vi "GEA_Brute_Force_SM0.vi"() -> ()   [LabVIEW 2009]
uses:
  <vilib>/Instr/_visa.llb/VISA Configure Serial Port (Instr).vi
panel:
  out "ACK":bool
  out "DataReturned":u8[](array[numeric]) format="%.0x"
  out "element":u8
  out "CRCRead":u8[](array[numeric]) format="%.0x"
  out "CRCArray":u8[](array[numeric]) format="%.0x"
  out "CRC Match":bool
  out "States Out":string
  out "error out":errorcluster
  in  "Source Address":u8=128 format="%.0x"
  in  "Command Data":u8[](array[numeric]) format="%02x"
  in  "Destination Address":u8=96 format="%.0x"
  in  "Command":u8(ring)=15 items=["CMD_WRITE_SETPOINTS", "RQST_NON_CRIT_VERSION", "RQST_CRIT_VERSION", "RQST_EEPROM_VERSION", "RQST_T2_RESISTANCE", "RQST_T3A_RESISTANCE", "RQST_T3B_RESISTANCE", "RQST_T4_RESISTANCE", "RQST_T5_RESISTANCE", "RQST_IDLB_RESISTANCE", "RQST_MODE_SELECT_RESISTANCE", "RQST_STATUS INFO", "RQST_SS_FAULT_COUNTS", "RQST_OTHER_FAULT_COUNTS", "CMD_CLEAR_FAULT_COUNTS", "RQST_HYPERTERM_OUTPUT_DATA", "RQST_READ_PERSONALITY", "RQST_DSM_OVERRIDE_STATUS", "RQST_STATUS_QUERY", "RQST_HEM_KWH_DATA", "RQST_SERVICE_ERROR_CODES", "RQST_OVERRIDE_STATUS", "CMD_CLEAR_OVERRIDE_STATUS", "CMD_CLEAR_ENERGY_USAGE_CTRS", "CMD_COMP_OFF", "CMD_UE_2_SECONDS", "CMD_LE_2_SECONDS", "CMD_COMP_ON", "CMD_HP_RUN_6MIN", "RQST_TEMP_RANGE", "RQST_VACATION_RANGE", "RQST_STD_ELEC_RANGE", "RQST_WATER_CAPACITY", "CMD_CANCEL_EEV_POSITION", "RQST_SUPPORTED_MODES", "CMD_CONTROL_FAN1", "CMD_EEV_POSITION", "CMD_SET_EEV_START_POSITION", "CMD_SET_EEV_STOP_POSITION", "CMD_UPDATE_DSM_LEVEL", "CMD_SET_PID_I_DENOMINATOR", "CMD_SET_PID_I_NUMERATOR", "RQST_DATA_FROM_MEMORY", "CMD_OVERRIDE_STATUS_CHANGED", "CMD_SET_PID_P_DENOMINATOR", "CMD_SET_PID_P_NUMERATOR", "CMD_SET_PID_RUN_SH_TARGET", "CMD_SET_PID_START_DWELL_TIME", "CMD_SET_PID_TRANSITION_TIME", "CMD_SET_PID_TRANS_SH_TARGET", "CMD_SET_PID_UPDATE_RATE", "RQST_DATA_FROM_DATA_FLASH", "CMD_DSM_OVERRIDES", "CMD_UPDATE_MODE", "CMD_UPDATE_SPECIAL_OPERATION", "CMD_SET_CURRENTS", "CMD_RESET_FILTER_TIMES", "CMD_TURN_ON_DLB", "RQST_PID_PARAMETERS", "CMD_CHECK_CRC", "CMD_ENTER_FACT_MODE", "CMD_RESET", "CMD_RESTORE_EEPROM_DEFAULTS"]
  out "Command":u8[](array[numeric])=[226, 96, 8, 128, 86, 123, 137, 227]
  in  "Send HEWH Cmd":bool
  in  "Write Rand":bool
  in  "Random Data":u8[](array[numeric]) format="%.0x"
  out "CRC 2":u8[](array[numeric])
  out "deleted portion 2":u8[](array[numeric])
  out "OldReadData":u8[](array[numeric])
  out "CRC Calc":u8[](array[numeric]) format="%.0x"
  in  "length":i32
  in  "Read Hyper":bool
  out "WriteOK":bool
  out "ReadArray":u8[](array[numeric]) format="%.0x"
  in  "Get Hyper Terminal Data":u8[](array[numeric])=[226, 96, 8, 128, 86, 123, 137, 227]
  in  "ComPort":refnum<visa-resource-name>="COM1"
  in  "OK":bool
  # "Special Character\tValue (Hexadecimal)\nESC\t0xE0  d224\nACK\t0xE1  d225\nSTX\t0xE2  d226\nETX\t0xE3  d227"
  # "[0] = Board Address\n\n[1] = UE\n[2] = LE\n[3] = Comp\n[4] = Fan\n[5] = Setpoint Deg F\n[6] = T2 Temp MSB (Deg F X 10)\n[7] = T2 Temp LSB (Deg F X 10)\n[8] = T3A Temp MSB (Deg F X 10)\n[9] = T3A Temp LSB (Deg F X 10)\n[10] = T3B Temp MSB (Deg F X 10)\n[11] = T3B Temp LSB (Deg F X 10)\n[12] = T4 Temp MSB (Deg F X 10)\n[13] = T4 Temp LSB (Deg F X 10)\n[14] = T5 Temp MSB (Deg F X 10)\n[15] = T5 Temp LSB (Deg F X 10)\n[16] = Current (AMPS X 10)\n[17] = Voltage MSB (Volts X 10)\n[18] = Voltage LSB (Volts X 10)\n[19] = EEV Position MSB (0-480)\n[20] = EEV Position LSB (0-480)"
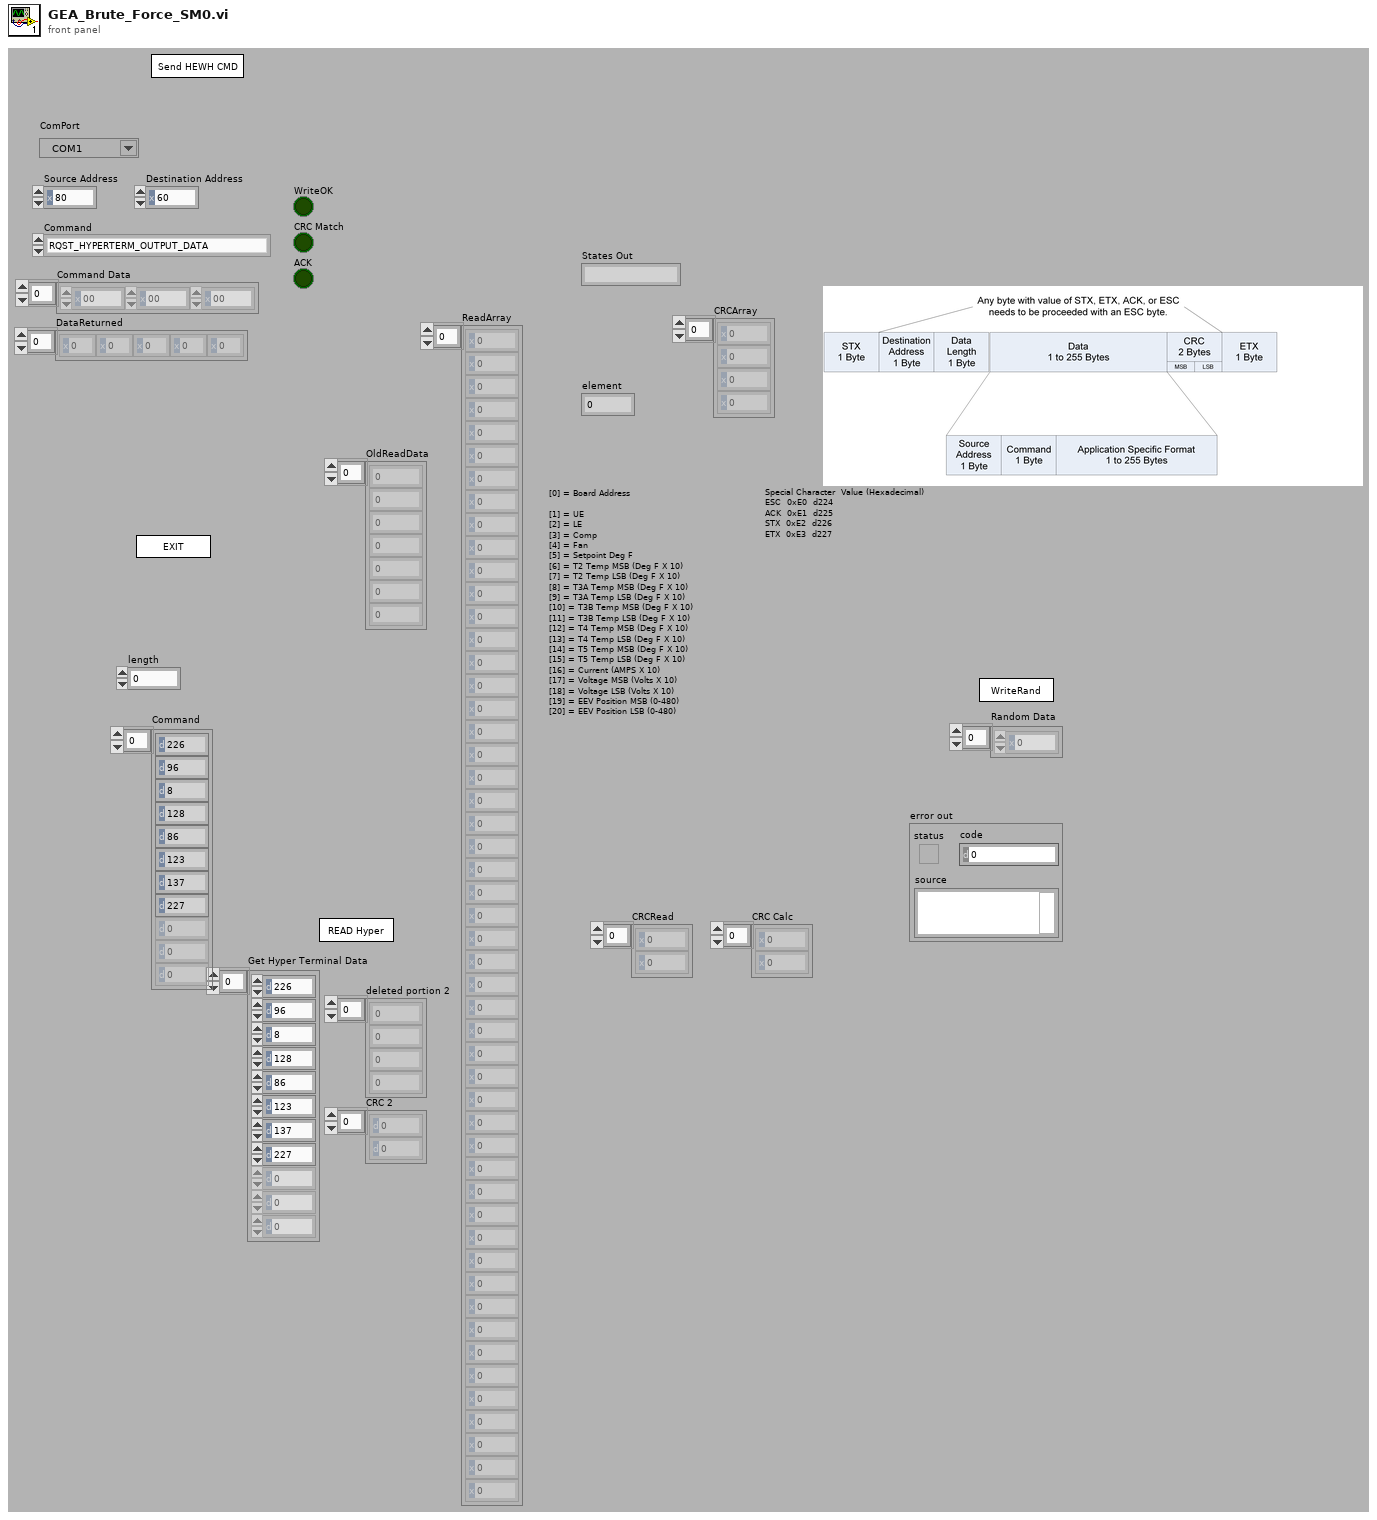
[diagram p1: front panel]
types:
  T1 = enum32{"invalid app kind", "Development System", "Run Time System", "Student Edition", "Embedded LabVIEW", "Evaluation", "Custom"}
  T2 = enum32{"Invalid", "Standard", "Closed", "Hidden", "Minimized", "Maximized"}
  T3 = cluster{"Core":cluster{"Current VI Reference":refnum<vi>, "Close Panel on Exit?":bool}, "ComPort":refnum<visa-resource-name>, "ReadArray":u8[], "CRCArray":u8[], "Bytes Remaining":u8, "CRCRead":u8[]}
  T4 = cluster{"Current VI Reference":refnum<vi>, "Close Panel on Exit?":bool}
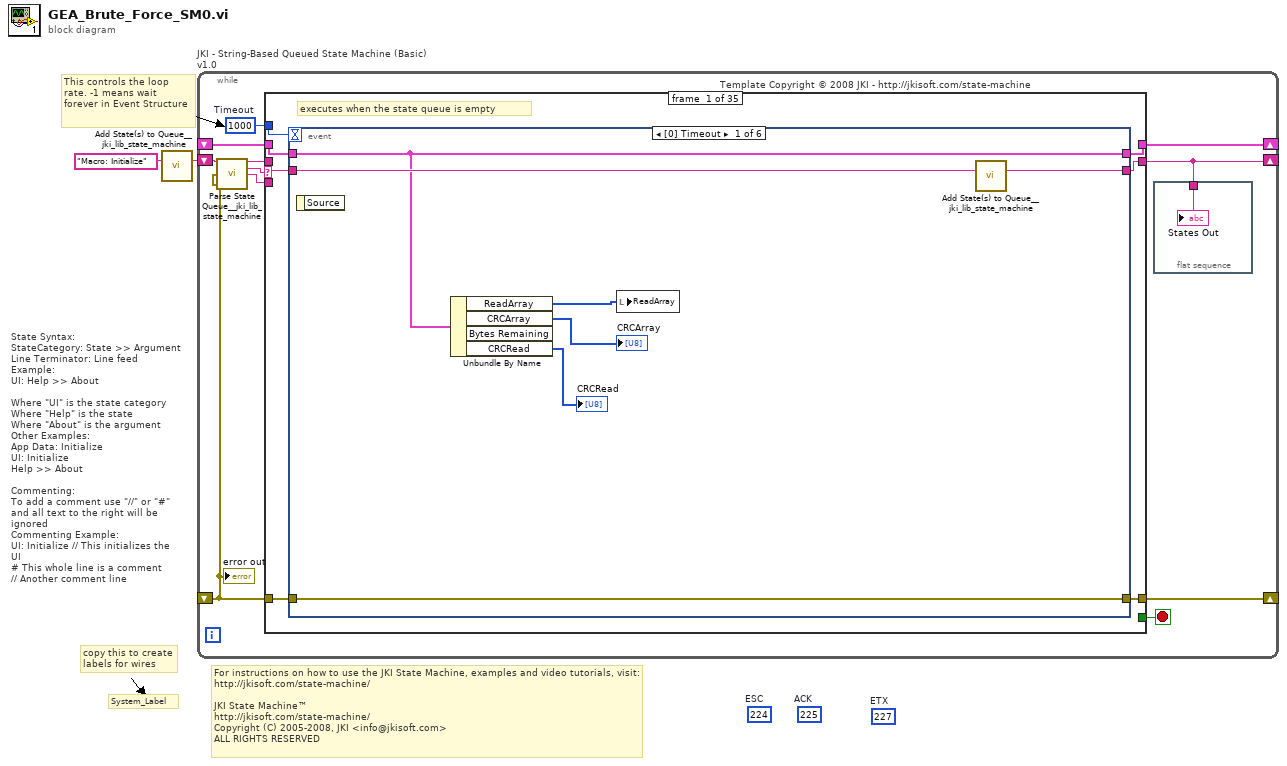
[diagram p0: block diagram]
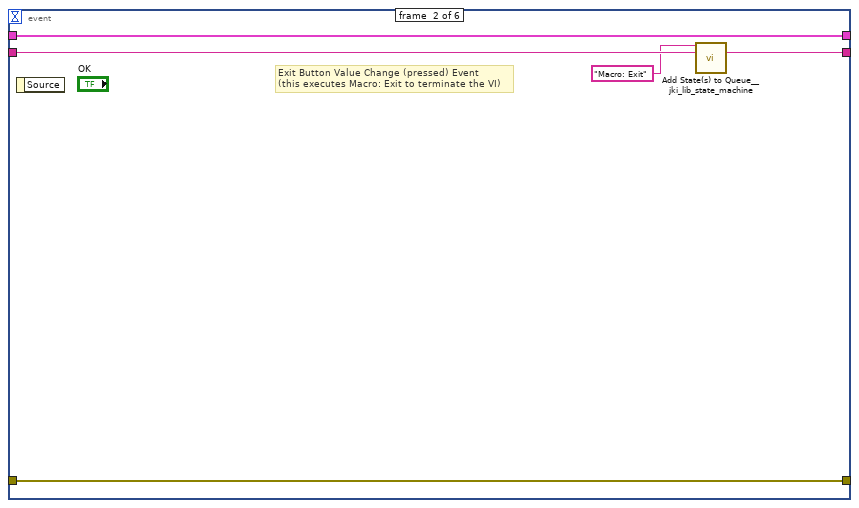
[diagram p2: hidden frame]
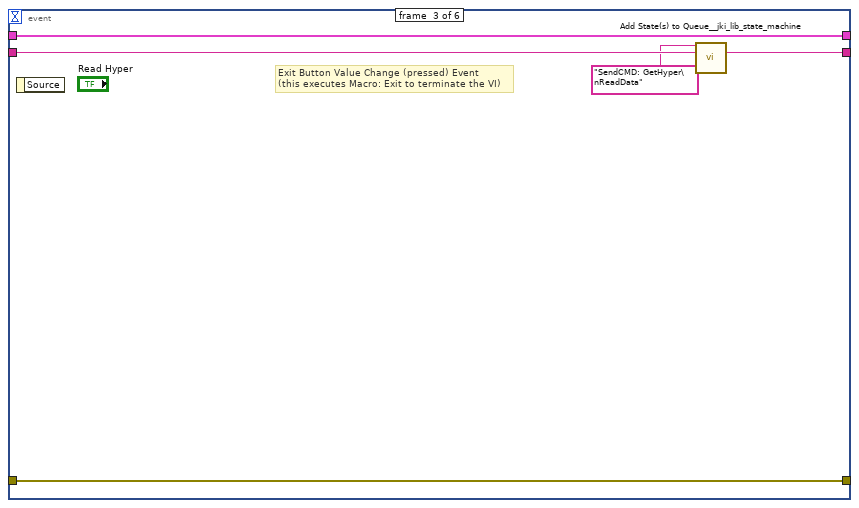
[diagram p3: hidden frame]
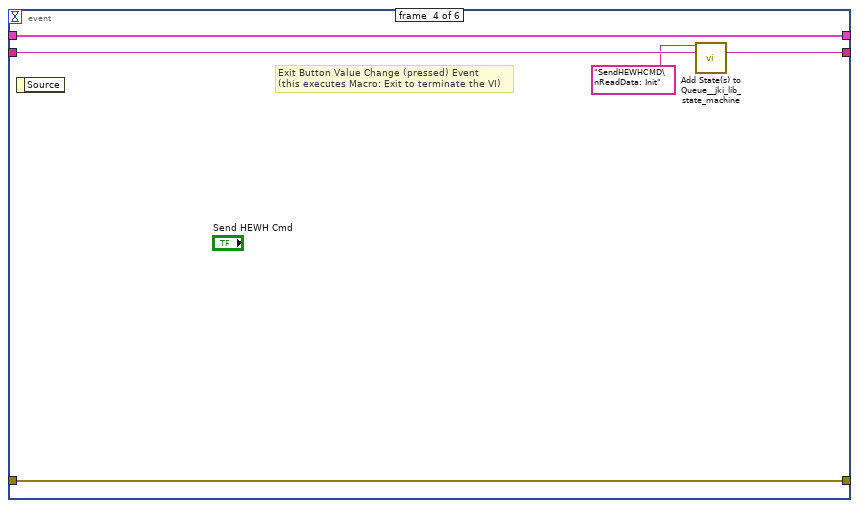
[diagram p4: hidden frame]
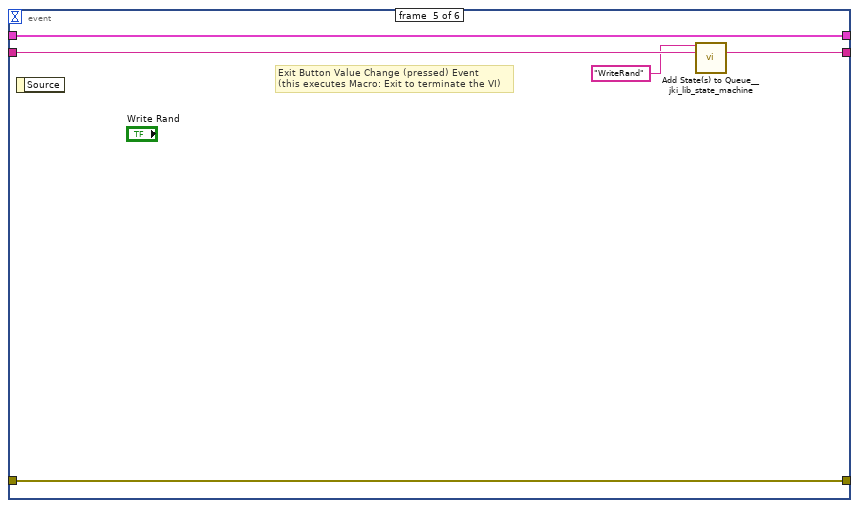
[diagram p5: hidden frame]
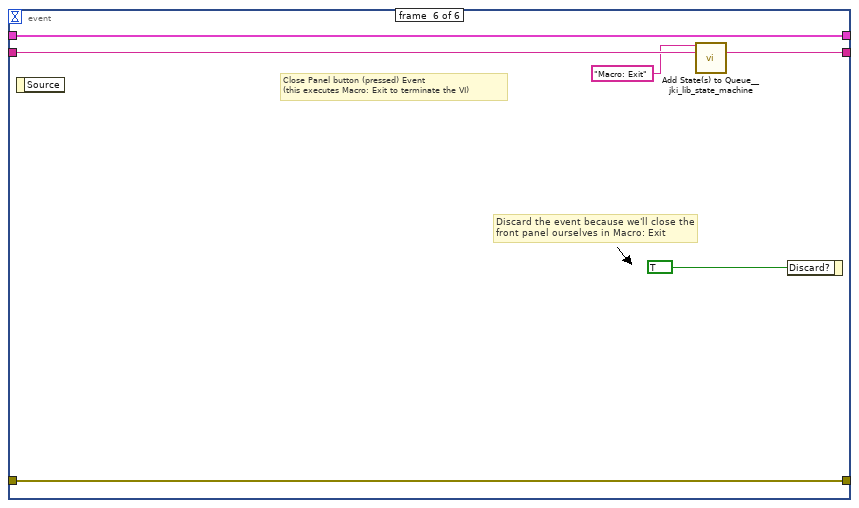
[diagram p6: hidden frame]
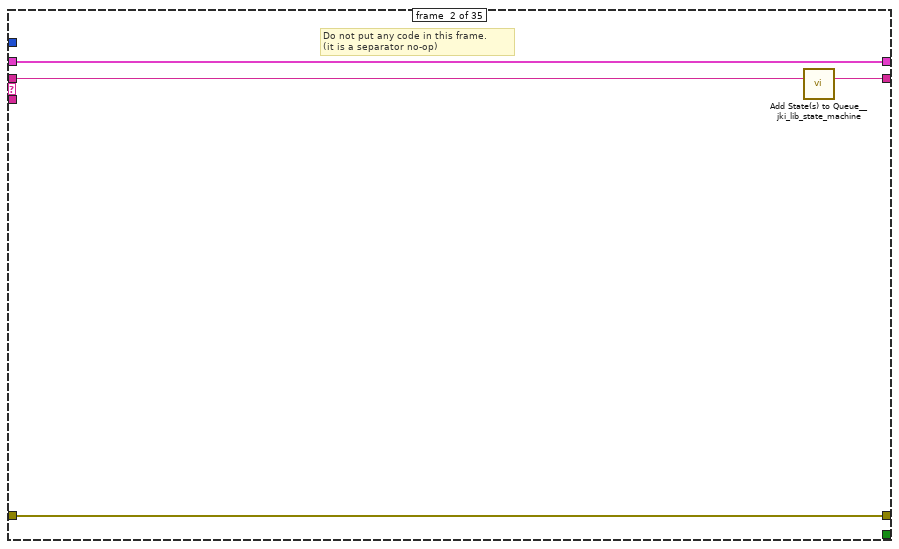
[diagram p7: hidden frame]
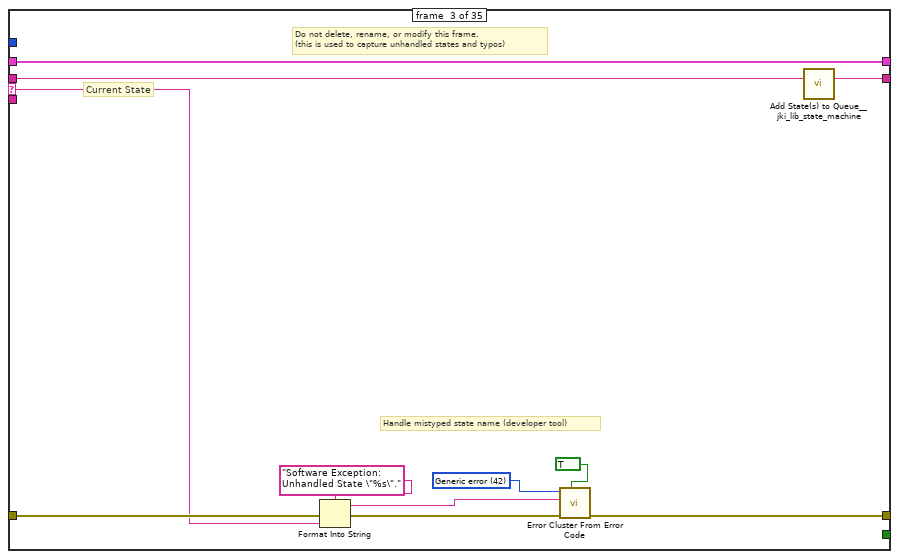
[diagram p8: hidden frame]
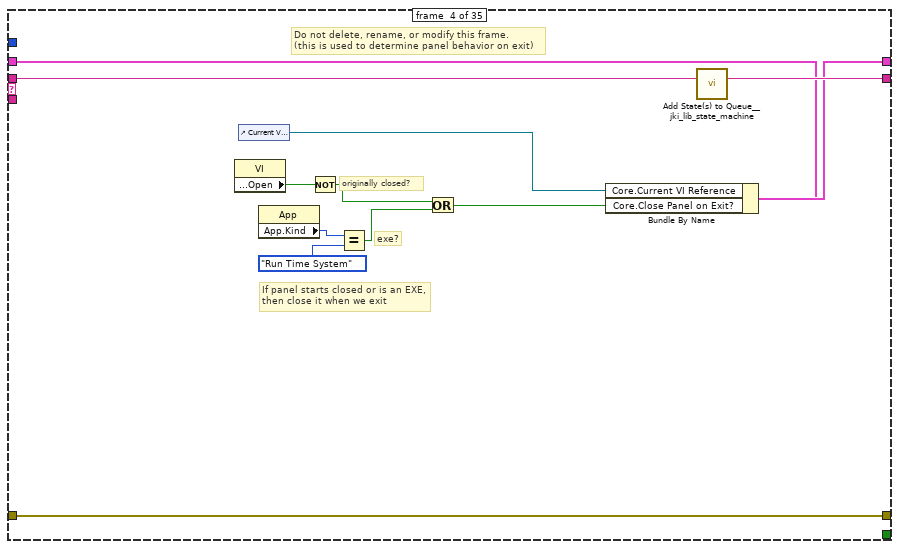
[diagram p9: hidden frame]
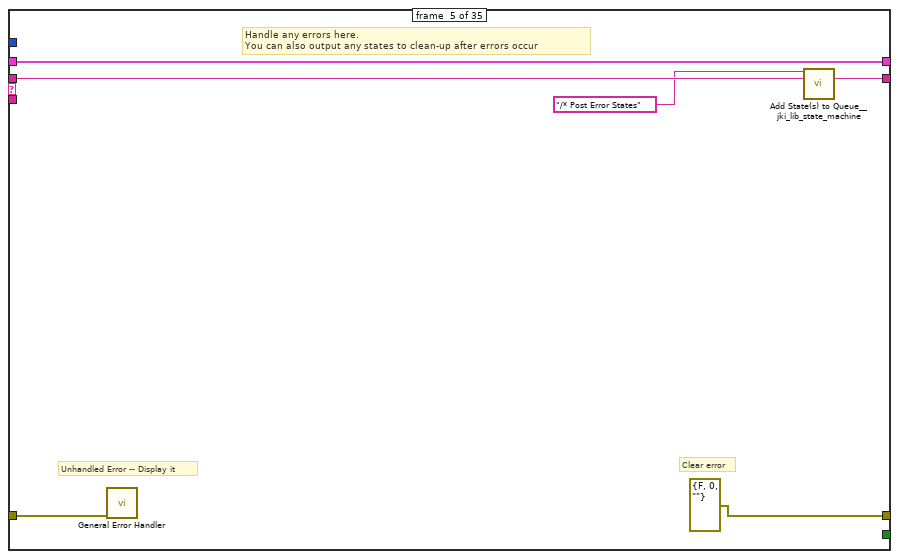
[diagram p10: hidden frame]
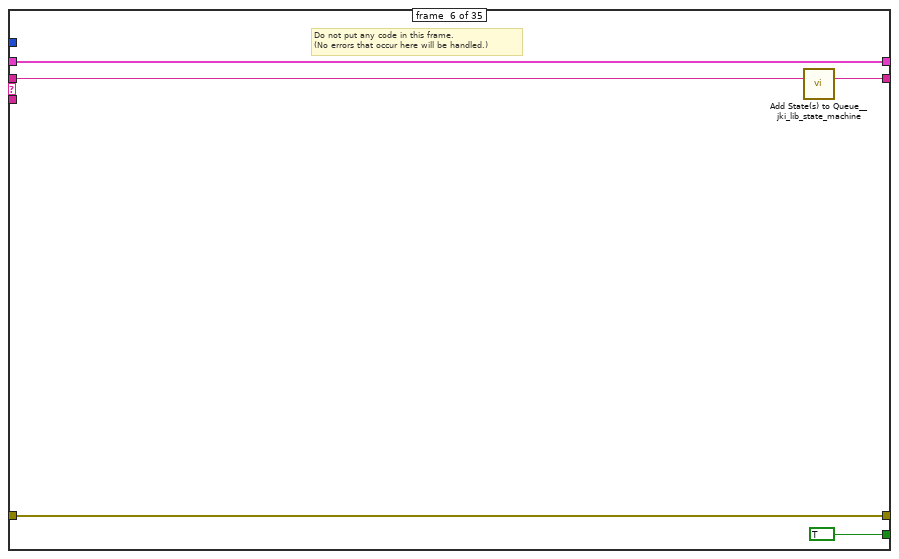
[diagram p11: hidden frame]
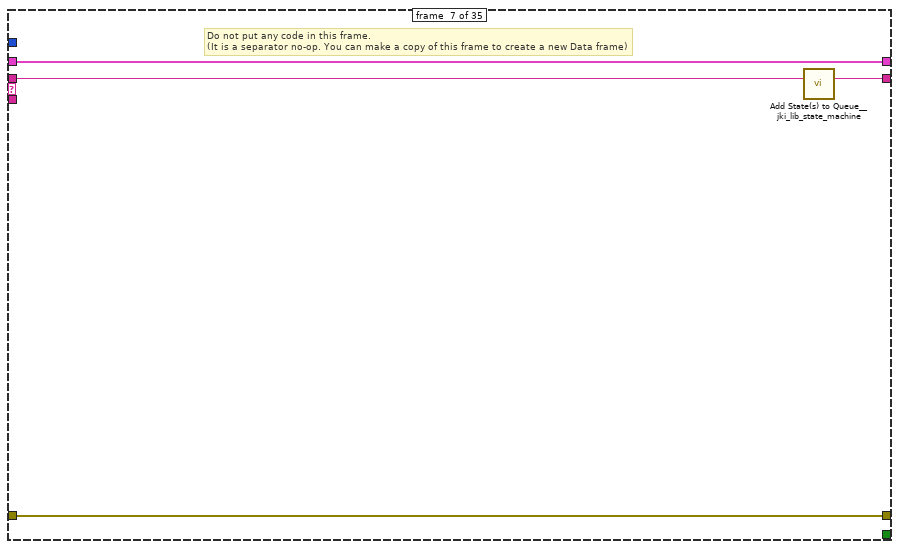
[diagram p12: hidden frame]
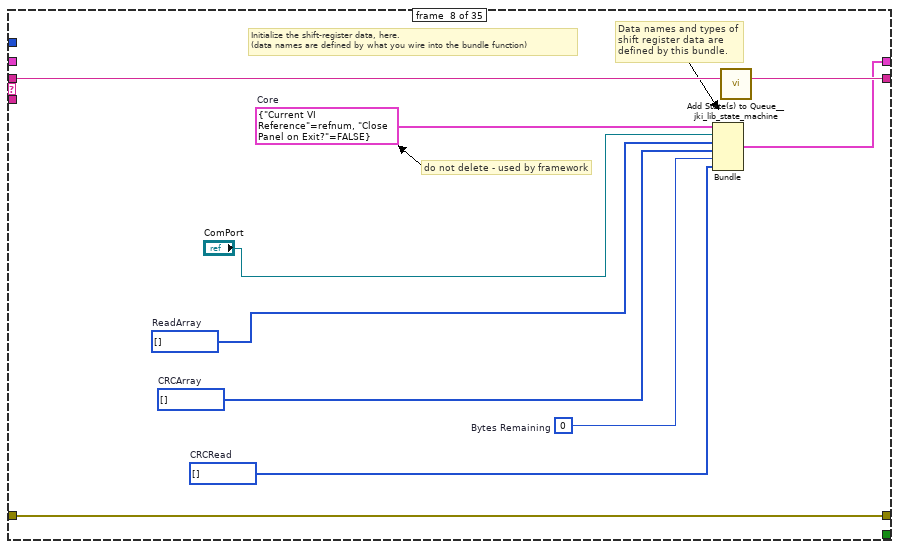
[diagram p13: hidden frame]
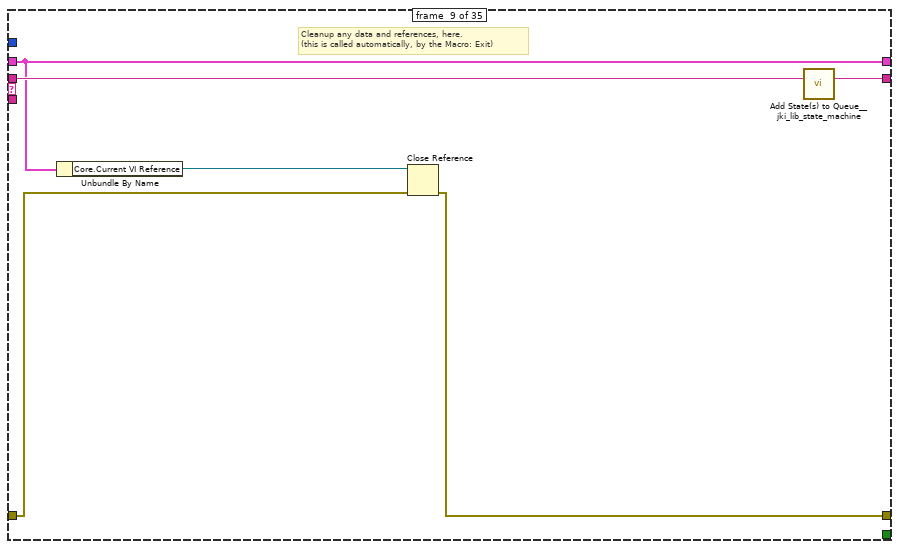
[diagram p14: hidden frame]
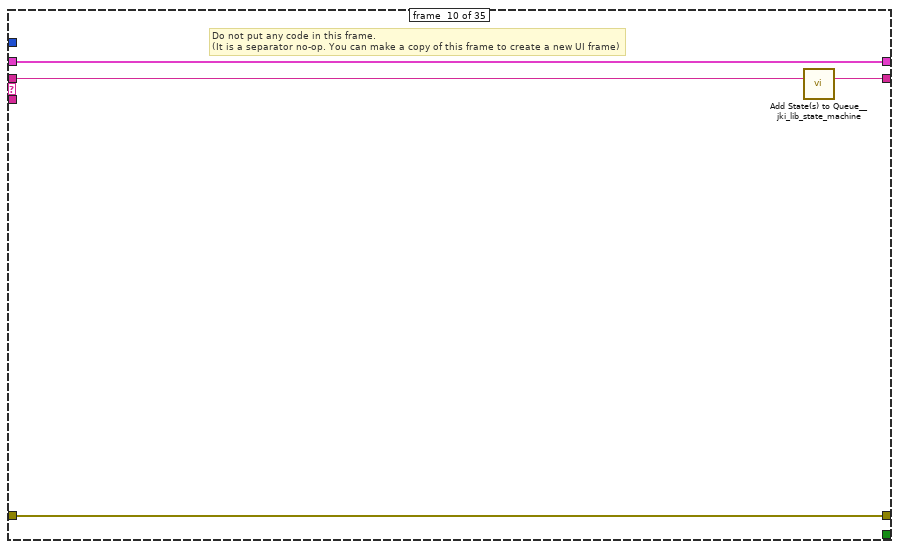
[diagram p15: hidden frame]
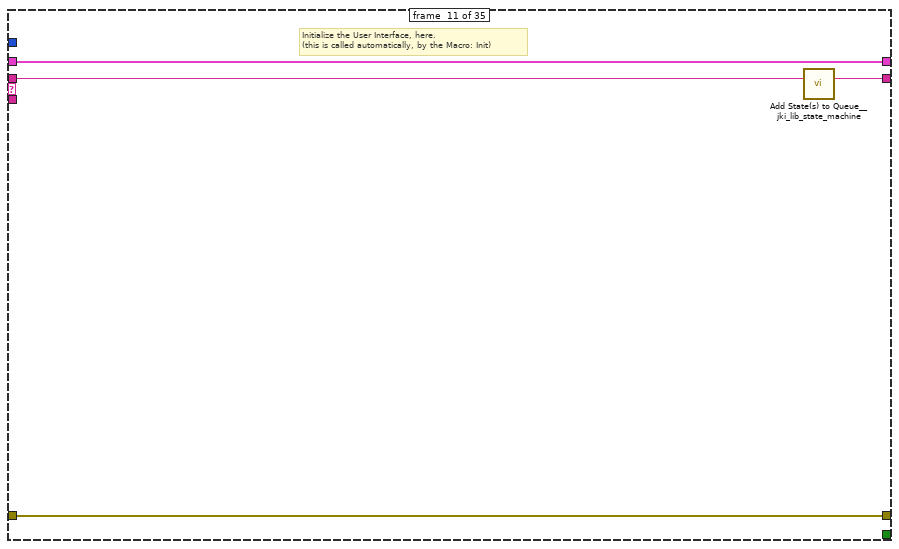
[diagram p16: hidden frame]
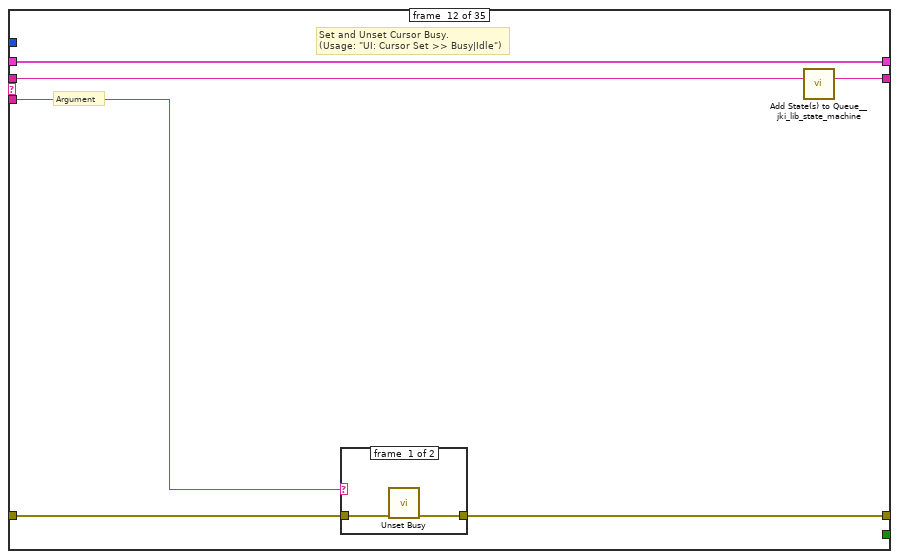
[diagram p17: hidden frame]
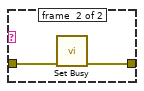
[diagram p18: hidden frame]
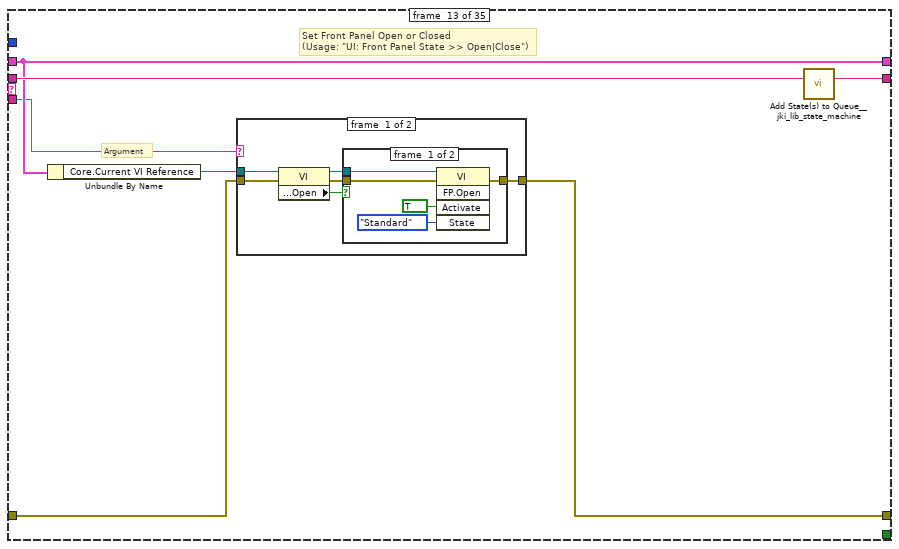
[diagram p19: hidden frame]
diagram:
  (unwired) u8 225  # ACK
  (unwired) u8 224  # ESC
  (unwired) u8 227  # ETX
  # "For instructions on how to use the JKI State Machine, examples and video tutorials, visit:\nhttp://jkisoft.com/state-machine/\n\nJKI State Machine™\nhttp://jkisoft.com/state-machine/\nCopyright (C) 2005-2008, JKI <info@jkisoft.com>\nALL RIGHTS RESERVED"
  # "State Syntax:\nStateCategory: State >> Argument\nLine Terminator: Line feed\nExample:\nUI: Help >> About\n\nWhere \"UI\" is the state category\nWhere \"Help\" is the state\nWhere \"About\" is the argument\nOther Examples:\nApp Data: Initialize\nUI: Initialize\nHelp >> About\n\nCommenting:\nTo add a comment use \"//\" or \"#\" and all text to the right will be ignored\nCommenting Example:\nUI: Initialize // This initializes the UI\n# This whole line is a comment\n// Another comment line"
  # "copy this to create labels for wires"
  # "This controls the loop rate. -1 means wait forever in Event Structure"
  # "System_Label"
  n1 = call <vilib>:"Add State(s) to Queue__jki_lib_state_machine.vi"("State(s) in (\"\")"="Macro: Initialize") -> ("States Out"=w2:string)  [unwired: 14 in]
  n2 = while "JKI - String-Based Queued State Machine (Basic) v1.0" {
    shift-right: [w6] -> _
    shift-left: _ -> [w5]
    shift-right: [w9] -> _
    shift-left: _ -> [w3]
    shift-right: [w8] -> _
    shift-left: w2 -> [w10]
    stop <- w7 stop-if-true
    w4 = 1000  # Timeout
    # "Template Copyright © 2008 JKI - http://jkisoft.com/state-machine"
    n3 = call <vilib>:"Parse State Queue__jki_lib_state_machine.vi"("State Queue"=w10, "Error In (no error)"=w3) -> ("Remaining States"=w12:string, "Current State"=w13:string, "Arguments"=w11:string)  [unwired: 11 in]
    n4 = case shown="\"ReadData\"" w13 {
      selector: w13 -> [_ _ w59 _ _ _ _ _ _ _ _ _ _ _ _ _ _ _ _ _ _ _ _ _ _ _ _ _ _ _ _ _ _ _ _]
      tunnel: w12 -> [w21 w58 w63 w81 w87 w92 w96 w106 w112 w116 w120 w126 w137 w163 w168 w178 w182 w200 w213 w247 w267 w287 w309 w316 w334 w365 w412 w456 w494 w528 w551 w575 w599 w613 w635]
      tunnel: w11 -> [_ _ _ _ _ _ _ _ _ _ _ w121 w131 _ _ _ _ _ _ _ _ _ _ _ _ _ _ _ _ _ _ _ _ _ _]
      tunnel: w5 -> [w19 w55 w61 w72 w84 w90 w93 _ w107 w113 w118 w124 w133 w160 w165 w175 w179 w187 w211 w245 w265 w284 w306 w313 w330 w362 w409 w453 w491 w526 w543 w570 w594 w608 w633]
      tunnel: [w18 w56 w65 w78 errorcluster {"status"=FALSE, "code"=0, "source"=""} ("error out") w89 w94 w103 w108 w114 w117 w122 w134 w161 w166 w176 w180 w189 w207 w241 w261 w285 w307 w314 w320 w354 w402 w448 w475 w512 w545 w565 w589 w611 w623] -> w9
      tunnel: w3 -> [w17 w56 w64 w78 w83 w89 w94 w103 w109 w114 w117 w123 w135 w161 w166 w176 w180 w184 w208 w242 w262 w285 w307 w314 w323 w356 w404 w449 w487 w522 w548 w568 w592 w611 w631]
      tunnel: [w20 w57 w62 w80 w86 w91 w95 w105 w111 w115 w119 w125 w136 w162 w167 w177 w181 w199 w212 w246 w266 w286 w308 w315 w333 w364 w411 w455 w493 w527 w550 w574 w598 w612 w634] -> w8
      tunnel: [_ _ _ _ _ TRUE _ _ _ _ _ _ _ _ _ _ _ _ _ _ _ _ _ _ _ _ _ _ _ _ _ _ _ _ _] -> w7
      tunnel: [w16 w55 w61 w79 w84 w90 w93 w104 w107 w113 w118 w124 w133 w160 w165 w175 w179 w186 w211 w245 w265 w284 w306 w312 w329 w361 w408 w452 w490 w525 w543 w569 w593 w607 w633] -> w6
      tunnel: w4 -> [w15 _ _ _ _ _ _ _ _ _ _ _ _ _ _ _ _ _ _ _ _ _ _ _ _ _ _ _ _ _ _ _ _ _ _]
      frame #0 {
        # "executes when the state queue is empty"
        n5 = event shown="[0] Timeout" {
          selector: _ -> [_ _ _ _ _ _]
          dyn-events: _ -> [_ _ _ _ _ _]
          timeout: w15 -> [_ _ _ _ _ _]
          tunnel: w21 -> [w28 w33 w38 w43 w48 w54]
          tunnel: [w27 w32 w37 w42 w47 w53] -> w20
          tunnel: w19 -> [w25 w30 w35 w40 w45 w51]
          tunnel: [w26 w31 w36 w41 w46 w52] -> w18
          tunnel: w17 -> [w26 w31 w36 w41 w46 w52]
          tunnel: [w25 w30 w35 w40 w45 w51] -> w16
          event #0 {
            n6 = event-data() -> ()  [unwired: 1 in, 1 out]
            n7 = Unbundle By Name(w25) -> ("ReadArray"=w24:u8[], "CRCArray"=→"CRCArray":u8[], "CRCRead"=→"CRCRead":u8[])  [unwired: 1 out]
            n8 = local write "ReadArray"(w24) -> ()
            n9 = call <vilib>:"Add State(s) to Queue__jki_lib_state_machine.vi"("State(s) in (\"\")"=w28) -> ("States Out"=w27:string)  [unwired: 14 in]
          }
          event #1 {
            # "Exit Button Value Change (pressed) Event\n(this executes Macro: Exit to terminate the VI)"
            n10 = event-data() -> ()  [unwired: 1 in, 1 out]
            n11 = call <vilib>:"Add State(s) to Queue__jki_lib_state_machine.vi"("State(s) in Front (\"\")"="Macro: Exit", "State(s) in (\"\")"=w33) -> ("States Out"=w32:string)  [unwired: 13 in]
          }
          event #2 {
            # "Exit Button Value Change (pressed) Event\n(this executes Macro: Exit to terminate the VI)"
            n12 = event-data() -> ()  [unwired: 1 in, 1 out]
            n13 = call <vilib>:"Add State(s) to Queue__jki_lib_state_machine.vi"("State(s) in Front (\"\")"="SendCMD: GetHyper\nReadData", "State(s) in (\"\")"=w38) -> ("States Out"=w37:string)  [unwired: 13 in]
          }
          event #3 {
            # "Exit Button Value Change (pressed) Event\n(this executes Macro: Exit to terminate the VI)"
            n14 = event-data() -> ()  [unwired: 1 in, 1 out]
            n15 = call <vilib>:"Add State(s) to Queue__jki_lib_state_machine.vi"("State(s) in Front (\"\")"="SendHEWHCMD\nReadData: Init", "State(s) in (\"\")"=w43) -> ("States Out"=w42:string)  [unwired: 13 in]
          }
          event #4 {
            # "Exit Button Value Change (pressed) Event\n(this executes Macro: Exit to terminate the VI)"
            n16 = event-data() -> ()  [unwired: 1 in, 1 out]
            n17 = call <vilib>:"Add State(s) to Queue__jki_lib_state_machine.vi"("State(s) in Front (\"\")"="WriteRand", "State(s) in (\"\")"=w48) -> ("States Out"=w47:string)  [unwired: 13 in]
          }
          event #5 {
            # "Discard the event because we'll close the front panel ourselves in Macro: Exit"
            # "Close Panel button (pressed) Event\n(this executes Macro: Exit to terminate the VI)"
            n18 = event-data() -> ()  [unwired: 1 in, 1 out]
            n19 = call <vilib>:"Add State(s) to Queue__jki_lib_state_machine.vi"("State(s) in Front (\"\")"="Macro: Exit", "State(s) in (\"\")"=w54) -> ("States Out"=w53:string)  [unwired: 13 in]
            n20 = event-data("Discard?"=TRUE) -> ()  [unwired: 1 in, 1 out]
          }
        }
      }
      frame #1 {
        # "Do not put any code in this frame.\n(it is a separator no-op)"
        n21 = call <vilib>:"Add State(s) to Queue__jki_lib_state_machine.vi"("State(s) in (\"\")"=w58) -> ("States Out"=w57:string)  [unwired: 14 in]
      }
      frame #2 {
        w68 = 42 items=["No error", "Argument error", "Memory is full", "Out of zone", "End of file", "File already open", "Generic file I/O error", "File not found", "File permission error", "Disk is full", "Duplicate path", "Too many files open", "System feature not enabled", "Resource file not found", "Cannot add resource", "Resource not found", "Image not found", "Image memory error", "Pen does not exist", "Config type invalid", "Config token not found", "Config parse error", "Config memory error", "Bad external code format", "Bad external code offset", "External code not present", "Null window", "Destroy window error", "Null menu", "Print aborted", "Bad print record", "Print driver error", "Windows error during printing", "Memory error during printing", "Print dialog error", "Generic print error", "Invalid device refnum", "Device not found", "Device parameter error", "Device unit error", "Cannot open device", "Device call aborted", "Generic error", "Cancelled by user", "Object ID too low", "Object ID too high", "Object not in heap", "Unknown heap", "Unknown object (invalid DefProc)", "Unknown object (DefProc not in table)", "Message out of range", "Invalid (null) method", "Unknown message", "Manager call not supported", "Bad address", "Network operation in progress", "Network operation timed out", "Connection is busy", "Network attribute not supported", "Network error", "Address in use", "System out of memory", "Connection aborted", "Connection refused", "Not connected", "Already connected", "Connection closed", "Initialization error (interapplication manager)", "Bad occurrence", "Wait on unbound occurrence handler", "Occurrence queue overflow", "Datalog type conflict", "Unused", "Unrecognized type (interapplication manager)", "Memory corrupt", "Failed to make temporary DLL", "Old CIN version", "Drag socket not found", "Failed to load drop-object", "Failed to register OLE object", "Failed to release OLE object", "Format specifier type mismatch", "Unknown format specifier", "Too few format specifiers", "Too many format specifiers", "Scan failed", "Newer CIN version", "Error converting to variant", "Runtime menu error", "Password tampered", "Variant attribute not found", "Incompatible variant data type", "Event data is not available", "Event Store is not present", "Occurrence is not found", "Event Queue is not created", "Event info is not available", "Refnum passed is NULL", "Error retrieving Class GUID", "Error retrieving CoClass GUID", "Error retrieving TypeLib GUID.", "Bad built application magic bytes.", "Specific driver is different from the specific driver associated with the Logical Name.", "There is no session opened to the class driver.", "Max Error", "MAX - Error with config objects", "MAX - Error loading configuration", "MAX - Group not supported"]
        # "Current State"
        # "Do not delete, rename, or modify this frame.\n(this is used to capture unhandled states and typos)"
        # "Handle mistyped state name (developer tool)"
        n22 = Format Into String(format string="Software Exception: Unhandled State \"%s\"." ("message"), error in=w64, w59) -> (resulting string=w67:string, error out=w66:errorcluster)  [unwired: 1 in]
        n23 = call <vilib>:"Error Cluster From Error Code.vi"("show call chain? (False)"=TRUE, "error in (no error)"=w66, "error message (\"\")"=w67, "error code (0)"=w68) -> ("error out"=w65:errorcluster)  [unwired: 5 in]
        n24 = call <vilib>:"Add State(s) to Queue__jki_lib_state_machine.vi"("State(s) in (\"\")"=w63) -> ("States Out"=w62:string)  [unwired: 14 in]
      }
      frame #3 {
        # "Do not delete, rename, or modify this frame.\n(this is used to determine panel behavior on exit)"
        # "originally closed?"
        # "exe?"
        # "If panel starts closed or is an EXE, then close it when we exit"
        n25 = property class="VI"() -> ("Front Panel.Open"=w77:bool)  [unwired: 2 in, 2 out]
        n26 = control-ref of="Current VI Reference"() -> (w70:refnum<vi>)
        n27 = property class="App"() -> ("App.Kind"=w76:T1)  [unwired: 2 in, 2 out]
        n28 = Not(x=w77) -> (.not. x?=w74:bool)
        n29 = Equal?(x=w76, y=T1."Run Time System" ("Application:Kind")) -> (x = y?=w73:bool)
        n30 = Or(x=w74, y=w73) -> (x .or. y?=w71:bool)
        n31 = Bundle By Name(cluster=w72, "Core.Current VI Reference"=w70, "Core.Close Panel on Exit?"=w71) -> (w79:T3)
        n32 = call <vilib>:"Add State(s) to Queue__jki_lib_state_machine.vi"("State(s) in (\"\")"=w81) -> ("States Out"=w80:string)  [unwired: 14 in]
      }
      frame #4 {
        # "Unhandled Error -- Display it"
        # "Handle any errors here.\nYou can also output any states to clean-up after errors occur"
        # "Clear error"
        n33 = call <vilib>:"General Error Handler.vi"("error in (no error)"=w83) -> ()  [unwired: 10 in, 5 out]
        n34 = call <vilib>:"Add State(s) to Queue__jki_lib_state_machine.vi"("State(s) in Front (\"\")"="/* Post Error States", "State(s) in (\"\")"=w87) -> ("States Out"=w86:string)  [unwired: 13 in]
      }
      frame #5 {
        # "Do not put any code in this frame.\n(No errors that occur here will be handled.)"
        n35 = call <vilib>:"Add State(s) to Queue__jki_lib_state_machine.vi"("State(s) in (\"\")"=w92) -> ("States Out"=w91:string)  [unwired: 14 in]
      }
      frame #6 {
        # "Do not put any code in this frame.\n(It is a separator no-op. You can make a copy of this frame to create a new Data frame)"
        n36 = call <vilib>:"Add State(s) to Queue__jki_lib_state_machine.vi"("State(s) in (\"\")"=w96) -> ("States Out"=w95:string)  [unwired: 14 in]
      }
      frame #7 {
        w97 = u8[] []  # CRCRead
        w98 = u8 0  # Bytes Remaining
        w99 = u8[] []  # CRCArray
        w100 = u8[] []  # ReadArray
        w102 = T4 {"Current VI Reference"=refnum, "Close Panel on Exit?"=FALSE}  # Core
        # "do not delete - used by framework"
        # "Data names and types of shift register data are defined by this bundle."
        # "Initialize the shift-register data, here.\n(data names are defined by what you wire into the bundle function)"
        n37 = Bundle("Core"=w102, "ComPort"="ComPort", "ReadArray"=w100, "CRCArray"=w99, "Bytes Remaining"=w98, "CRCRead"=w97) -> (w104:T3)  [unwired: 1 in]
        n38 = call <vilib>:"Add State(s) to Queue__jki_lib_state_machine.vi"("State(s) in (\"\")"=w106) -> ("States Out"=w105:string)  [unwired: 14 in]
      }
      frame #8 {
        # "Cleanup any data and references, here.\n(this is called automatically, by the Macro: Exit)"
        n39 = Unbundle By Name(w107) -> ("Core.Current VI Reference"=w110:refnum<vi>)
        n40 = Close Reference(reference=w110, error in (no error)=w109) -> (error out=w108:errorcluster)
        n41 = call <vilib>:"Add State(s) to Queue__jki_lib_state_machine.vi"("State(s) in (\"\")"=w112) -> ("States Out"=w111:string)  [unwired: 14 in]
      }
      frame #9 {
        # "Do not put any code in this frame.\n(It is a separator no-op. You can make a copy of this frame to create a new UI frame)"
        n42 = call <vilib>:"Add State(s) to Queue__jki_lib_state_machine.vi"("State(s) in (\"\")"=w116) -> ("States Out"=w115:string)  [unwired: 14 in]
      }
      frame #10 {
        # "Initialize the User Interface, here.\n(this is called automatically, by the Macro: Init)"
        n43 = call <vilib>:"Add State(s) to Queue__jki_lib_state_machine.vi"("State(s) in (\"\")"=w120) -> ("States Out"=w119:string)  [unwired: 14 in]
      }
      frame #11 {
        # "Argument"
        # "Set and Unset Cursor Busy.\n(Usage: \"UI: Cursor Set >> Busy|Idle\")"
        n44 = case shown="\"Idle\", Default" w121 {
          tunnel: w123 -> [w128 w130]
          tunnel: [w127 w129] -> w122
          frame #0 {
            n45 = call <vilib>:"Unset Busy.vi"("error in (no error)"=w128) -> ("error out"=w127:errorcluster)  [unwired: 10 in]
          }
          frame #1 {
            n46 = call <vilib>:"Set Busy.vi"("error in (no error)"=w130) -> ("error out"=w129:errorcluster)  [unwired: 9 in, 1 out]
          }
        }
        n47 = call <vilib>:"Add State(s) to Queue__jki_lib_state_machine.vi"("State(s) in (\"\")"=w126) -> ("States Out"=w125:string)  [unwired: 14 in]
      }
      frame #12 {
        # "Argument"
        # "Set Front Panel Open or Closed\n(Usage: \"UI: Front Panel State >> Open|Close\")"
        n48 = Unbundle By Name(w133) -> ("Core.Current VI Reference"=w132:refnum<vi>)
        n49 = case shown="\"Open\", Default" w131 {
          tunnel: w135 -> [w141 w154]
          tunnel: [w143 w155] -> w134
          tunnel: w132 -> [w142 w152]
          frame #0 {
            n50 = property class="VI"(reference=w142, error in=w141) -> (reference out=w139:refnum<vi>, error out=w140:errorcluster, "Front Panel.Open"=w138:bool)
            n51 = case shown="False" w138 {
              tunnel: [w146 w149] -> w143
              tunnel: w140 -> [w145 w149]
              tunnel: w139 -> [w144 _]
              frame #0 {
                n52 = invoke class="VI" method="FP.Open"(reference=w144, error in=w145, "Activate"=TRUE, "State"=T2."Standard") -> (error out=w146:errorcluster)  [unwired: 1 in, 4 out]
              }
              frame #1 {
              }
            }
          }
          frame #1 {
            n53 = property class="VI"(reference=w152, error in=w154) -> (reference out=w151:refnum<vi>, error out=w153:errorcluster, "Front Panel.Open"=w150:bool)
            n54 = case shown="True" w150 {
              tunnel: [w156 w159] -> w155
              tunnel: w153 -> [w156 w158]
              tunnel: w151 -> [_ w157]
              frame #0 {
              }
              frame #1 {
                n55 = invoke class="VI" method="FP.Close"(reference=w157, error in=w158) -> (error out=w159:errorcluster)  [unwired: 1 in, 2 out]
              }
            }
          }
        }
        n56 = call <vilib>:"Add State(s) to Queue__jki_lib_state_machine.vi"("State(s) in (\"\")"=w137) -> ("States Out"=w136:string)  [unwired: 14 in]
      }
      frame #13 {
        # "Do not put any code in this frame.\n(It is a separator no-op. You can make a copy of this frame to create a new Macro frame)"
        n57 = call <vilib>:"Add State(s) to Queue__jki_lib_state_machine.vi"("State(s) in (\"\")"=w163) -> ("States Out"=w162:string)  [unwired: 14 in]
      }
      frame #14 {
        w164 = "Data: Initialize\nInitialize Core Data\nUI: Initialize\nUI: Front Panel State >> Open\nInit_Serial"  # Data: Initialize Initialize Core Data UI: Initialize UI: Front Panel State >> Open Init_Serial
        # "Initialization Macro\n(This is called once, when the VI starts)"
        n58 = call <vilib>:"Add State(s) to Queue__jki_lib_state_machine.vi"("State(s) in Front (\"\")"=w164, "State(s) in (\"\")"=w168) -> ("States Out"=w167:string)  [unwired: 13 in]
      }
      frame #15 {
        # "Exit Macro\n(This is called once, when the VI exits)"
        n59 = Unbundle By Name(w175) -> ("Core.Close Panel on Exit?"=w174:bool)
        n60 = Select(t="UI: Front Panel State >> Close", s=w174, f="") -> (s? t:f=w171:string)
        n61 = call <vilib>:"Add State(s) to Queue__jki_lib_state_machine.vi"("State(s) in (\"\")"=w171, "State(s) at Back (\"\")"="Data: Cleanup\nExit") -> ("States Out"=w169:string)  [unwired: 13 in]
        n62 = call <vilib>:"Add State(s) to Queue__jki_lib_state_machine.vi"("State(s) in Front (\"\")"=w169, "State(s) in (\"\")"=w178) -> ("States Out"=w177:string)  [unwired: 13 in]
      }
      frame #16 {
        # "Template Separator\n(You can make a copy of, or modify, this frame)"
        n63 = call <vilib>:"Add State(s) to Queue__jki_lib_state_machine.vi"("State(s) in (\"\")"=w182) -> ("States Out"=w181:string)  [unwired: 14 in]
      }
      frame #17 {
        w197 = u16 0 items=["None", "XON/XOFF", "RTS/CTS", "XON/XOFF & RTS/CTS", "DTR/DSR", "XON/XOFF & DTR/DSR"] ("flow control (0:none)")
        w196 = u16 10 items=["1.0"=10, "1.5"=15, "2.0"=20] ("stop bits (10: 1 bit)")
        # "Your code here.\n(You can make a copy of, or modify, this frame)"
        n64 = Unbundle By Name(w187) -> ("ComPort"=w185:refnum<visa-resource-name>)
        n65 = VISA Close(VISA resource name=w185, error in (no error)=w184) -> (error out=w183:errorcluster)
        n66 = call-poly "VISA Configure Serial Port"("VISA resource name"=w185, "timeout (10sec)"=u32 150, "Enable Termination\nChar (T)"=FALSE ("Enable Termination\nChar (T)"), "baud rate (9600)"=u32 19200, "data bits (8)"=u16 8, "parity (0:none)"=enum16{"None", "Odd", "Even", "Mark", "Space"}."None", "error in (no error)"=w183, "stop bits (10: 1 bit)"=w196, "flow control (0:none)"=w197) -> ("VISA resource name out"=w192:refnum<visa-resource-name>, "error out"=w190:errorcluster)  [unwired: 5 in]
        n67 = VISA Clear(VISA resource name=w192, error in (no error)=w190) -> (VISA resource name out=w188:refnum<visa-resource-name>, error out=w189:errorcluster)
        n68 = Bundle By Name(cluster=w187, "ComPort"=w188) -> (w186:T3)
        n69 = call <vilib>:"Add State(s) to Queue__jki_lib_state_machine.vi"("State(s) in (\"\")"=w200) -> ("States Out"=w199:string)  [unwired: 14 in]
      }
      frame #18 {
        n70 = Unbundle By Name(w211) -> ("ComPort"=w210:refnum<visa-resource-name>)
        n71 = for {
          tunnel: w210 -> [w224]
          tunnel: "Get Hyper Terminal Data" -> [w220] mode=indexing
          tunnel: [w217] -> w209 mode=indexing
          shift-right: [w216] -> w207
          shift-left: w208 -> [w215]
          n72 = Build Array(w220) -> (w221:u8[])
          n73 = Byte Array To String(unsigned byte array=w221) -> (string=w218:string)
          n74 = VISA Write(VISA resource name=w224, write buffer=w218, error in (no error)=w215) -> (VISA resource name out=w223:refnum<visa-resource-name>, error out=w214:errorcluster)  [unwired: 1 out]
          n75 = VISA Read(VISA resource name=w223, byte count=u32 1, error in (no error)=w214) -> (read buffer=w219:string, error out=w216:errorcluster)  [unwired: 2 out]
          n76 = Equal?(x=w218, y=w219) -> (x = y?=w217:bool)
        }
        n77 = Delete From Array(array="Get Hyper Terminal Data", length=4, index=1) -> (deleted portion=w205:u8[])  [unwired: 1 out]
        "deleted portion 2" <- w205
        n78 = call "crc16-ccitt (x1021).vi"("unsigned byte array"=w205) -> ("CRC"=→"CRC 2":u8[])  [unwired: 9 in, 1 out]
        n79 = And Array Elements(Boolean array=w209) -> (logical AND=→"WriteOK":bool)
        n80 = call <vilib>:"Add State(s) to Queue__jki_lib_state_machine.vi"("State(s) in (\"\")"=w213) -> ("States Out"=w212:string)  [unwired: 14 in]
      }
      frame #19 {
        w227 = u8 227  # ETX
        w230 = u8 226  # STX
        # "Your code here.\n(You can make a copy of, or modify, this frame)"
        n81 = Unbundle By Name(w245) -> ("ComPort"=w244:refnum<visa-resource-name>)
        n82 = call "HEWH_DSM_CMD.vi"("Command"="Command") -> ("CMD Array"=w232:u8[])  [unwired: 10 in]
        n83 = Array Size(array=w232) -> (size(s)=w238:i32)
        n84 = Array Size(array="Command Data") -> (size(s)=w236:i32)
        n85 = Compound Arithmetic op=ADD(7 ("x"), w238, w236) -> (w234:i32)
        n86 = To Unsigned Byte Integer(number=w234) -> (unsigned 8bit integer=w235:u8)
        n87 = Build Array (concatenate)("Destination Address", w235, "Source Address", w232, "Command Data") -> (w229:u8[])
        n88 = call "crc16-ccitt (x1021).vi"("unsigned byte array"=w229) -> ("CRC"=w228:u8[])  [unwired: 9 in, 1 out]
        n89 = Build Array (concatenate)(w230, w229, w228, w227) -> (w226:u8[])
        "Command" <- w226
        n90 = for {
          tunnel: w244 -> [w258]
          tunnel: w226 -> [w254] mode=indexing
          tunnel: [w251] -> w243 mode=indexing
          shift-right: [w250] -> w241
          shift-left: w242 -> [w249]
          n91 = Build Array(w254) -> (w255:u8[])
          n92 = Byte Array To String(unsigned byte array=w255) -> (string=w252:string)
          n93 = VISA Write(VISA resource name=w258, write buffer=w252, error in (no error)=w249) -> (VISA resource name out=w257:refnum<visa-resource-name>, error out=w248:errorcluster)  [unwired: 1 out]
          n94 = VISA Read(VISA resource name=w257, byte count=u32 1, error in (no error)=w248) -> (read buffer=w253:string, error out=w250:errorcluster)  [unwired: 2 out]
          n95 = Equal?(x=w252, y=w253) -> (x = y?=w251:bool)
        }
        n96 = And Array Elements(Boolean array=w243) -> (logical AND=w225:bool)
        n97 = call <vilib>:"Add State(s) to Queue__jki_lib_state_machine.vi"("State(s) in (\"\")"=w247) -> ("States Out"=w246:string)  [unwired: 14 in]
        n98 = local write "WriteOK"(w225) -> ()
      }
      frame #20 {
        # "Your code here.\n(You can make a copy of, or modify, this frame)"
        n99 = Unbundle By Name(w265) -> ("ComPort"=w264:refnum<visa-resource-name>)
        n100 = for {
          tunnel: w264 -> [w278]
          tunnel: "Random Data" -> [w274] mode=indexing
          tunnel: [w271] -> w263 mode=indexing
          shift-right: [w270] -> w261
          shift-left: w262 -> [w269]
          n101 = Build Array(w274) -> (w275:u8[])
          n102 = Byte Array To String(unsigned byte array=w275) -> (string=w272:string)
          n103 = VISA Write(VISA resource name=w278, write buffer=w272, error in (no error)=w269) -> (VISA resource name out=w277:refnum<visa-resource-name>, error out=w268:errorcluster)  [unwired: 1 out]
          n104 = VISA Read(VISA resource name=w277, byte count=u32 1, error in (no error)=w268) -> (read buffer=w273:string, error out=w270:errorcluster)  [unwired: 2 out]
          n105 = Equal?(x=w272, y=w273) -> (x = y?=w271:bool)
        }
        n106 = And Array Elements(Boolean array=w263) -> (logical AND=w259:bool)
        n107 = local write "WriteOK"(w259) -> ()
        n108 = call <vilib>:"Add State(s) to Queue__jki_lib_state_machine.vi"("State(s) in (\"\")"=w267) -> ("States Out"=w266:string)  [unwired: 14 in]
      }
      frame #21 {
        # "Your code here.\n(You can make a copy of, or modify, this frame)"
        n109 = Unbundle By Name(w284) -> ("ComPort"=w283:refnum<visa-resource-name>)
        n110 = stacked-sequence {
          tunnel: w283 -> [w298]
          tunnel: [w289] -> w281
          tunnel: u8[] [] -> [w288]
          frame #0 {
            n111 = while {
              shift-right: [w300] -> w293
              shift-left: w288 -> [w302]
              tunnel: w298 -> [w301]
              stop <- w299 stop-if-true
              n112 = VISA Read(VISA resource name=w301, byte count=u32 1) -> (read buffer=w304:string, error out=w299:errorcluster)  [unwired: 1 in, 2 out]
              n113 = String To Byte Array(string=w304) -> (unsigned byte array=w303:u8[])
              n114 = Build Array (concatenate)(w302, w303) -> (w300:u8[])
            }
            "ReadArray" <- w293
            n115 = Delete From Array(array=w293, length="length", index=2) -> (deleted portion=w297:u8[])  [unwired: 1 out]
            "OldReadData" <- w297
            n116 = call "crc16-ccitt (x1021).vi"("unsigned byte array"=w297) -> ("CRC"=w290:u8[])  [unwired: 9 in, 1 out]
            "CRC Calc" <- w290
            n117 = Delete From Array(array=w293, length=2, index=26) -> (deleted portion=w291:u8[])  [unwired: 1 out]
            n118 = Equal?(x=w291, y=w290) -> (x = y?=w289:bool)
          }
        }
        n119 = Select(t="", s=w281, f="SendCMD: GetHyper\nReadData") -> ()  [unwired: 1 out]
        n120 = call <vilib>:"Add State(s) to Queue__jki_lib_state_machine.vi"("State(s) in (\"\")"=w287) -> ("States Out"=w286:string)  [unwired: 14 in]
      }
      frame #22 {
        # "Template Separator\n(You can make a copy of, or modify, this frame)"
        n121 = call <vilib>:"Add State(s) to Queue__jki_lib_state_machine.vi"("State(s) in (\"\")"=w309) -> ("States Out"=w308:string)  [unwired: 14 in]
      }
      frame #23 {
        w310 = u8[] [] ("ReadArray")
        # "Your code here.\n(You can make a copy of, or modify, this frame)"
        n122 = Bundle By Name(cluster=w313, "ReadArray"=w310, "CRCArray"=w310) -> (w312:T3)
        n123 = local write "ReadArray"(w310) -> ()
        n124 = call <vilib>:"Add State(s) to Queue__jki_lib_state_machine.vi"("State(s) in Front (\"\")"="ReadData: ACK" ("State(s) in Front (\"\")"), "State(s) in (\"\")"=w316) -> ("States Out"=w315:string)  [unwired: 13 in]
      }
      frame #24 {
        w318 = u8 225  # ACK
        # "Your code here.\n(You can make a copy of, or modify, this frame)"
        n125 = Unbundle By Name(w330) -> ("ComPort"=w332:refnum<visa-resource-name>, "ReadArray"=w317:u8[])
        n126 = local write "ReadArray"(w317) -> ()
        n127 = VISA Read(VISA resource name=w332, byte count=u32 1, error in (no error)=w323) -> (read buffer=w327:string, error out=w321:errorcluster)  [unwired: 2 out]
        n128 = String To Byte Array(string=w327) -> (unsigned byte array=w326:u8[])
        n129 = Index Array(array=w326, index=0) -> (element=w324:u8)
        n130 = Build Array (concatenate)(w317, w326) -> (w331:u8[])
        n131 = Equal?(x=w324, y=w318) -> (x = y?=w322:bool)
        n132 = Bundle By Name(cluster=w330, "ReadArray"=w331) -> (w329:T3)
        n133 = case shown="False" w322 {
          tunnel: w321 -> [w338 w340]
          tunnel: [w336 w340] -> w320
          tunnel: ["ReadData: Rest" ("State(s) in Front (\"\")") "ReadData: STX" ("State(s) in Front (\"\")")] -> w319
          frame #0 {
            n134 = call <vilib>:"Merge Errors.vi"("error in 2 (no error)"=errorcluster {"status"=TRUE, "code"=7000, "source"="No ACK"}, "error in 1 (no error)"=w338) -> ("error out"=w336:errorcluster)  [unwired: 5 in]
          }
          frame #1 {
          }
        }
        n135 = call <vilib>:"Add State(s) to Queue__jki_lib_state_machine.vi"("State(s) in Front (\"\")"=w319, "State(s) in (\"\")"=w334) -> ("States Out"=w333:string)  [unwired: 13 in]
      }
      frame #25 {
        w349 = u8 224  # ESC
        # "Your code here.\n(You can make a copy of, or modify, this frame)"
        n136 = Unbundle By Name(w362) -> ("ComPort"=w342:refnum<visa-resource-name>, "ReadArray"=w341:u8[])
        n137 = VISA Read(VISA resource name=w342, byte count=u32 1, error in (no error)=w356) -> (read buffer=w359:string, error out=w344:errorcluster)  [unwired: 2 out]
        n138 = String To Byte Array(string=w359) -> (unsigned byte array=w346:u8[])
        n139 = Index Array(array=w346, index=0) -> (element=w351:u8)
        n140 = local write "ReadArray"(w341) -> ()
        n141 = Equal?(x=w351, y=w349) -> (x = y?=w348:bool)
        n142 = case shown="False" w348 {
          tunnel: [w368 w369] -> w347
          tunnel: w346 -> [w368 w376]
          tunnel: [w367 w370] -> w345
          tunnel: w341 -> [w367 w377]
          tunnel: w344 -> [w366 w373]
          tunnel: [w366 w372] -> w343
          tunnel: w342 -> [_ w371]
          frame #0 {
          }
          frame #1 {
            n143 = VISA Read(VISA resource name=w371, byte count=u32 1, error in (no error)=w373) -> (read buffer=w375:string, error out=w372:errorcluster)  [unwired: 2 out]
            n144 = String To Byte Array(string=w375) -> (unsigned byte array=w369:u8[])
            n145 = Build Array (concatenate)(w377, w376) -> (w370:u8[])
          }
        }
        n146 = local read "Source Address"() -> (w352:u8)
        n147 = Build Array (concatenate)(w345, w347) -> (w363:u8[])
        n148 = Index Array(array=w347, index=0) -> (element=w357:u8)
        n149 = Equal?(x=w357, y=w352) -> (x = y?=w355:bool)
        n150 = Bundle By Name(cluster=w362, "ReadArray"=w363, "CRCArray"=w347) -> (w361:T3)
        n151 = case shown="True" w355 {
          tunnel: w343 -> [w381 w383]
          tunnel: [w379 w383] -> w354
          tunnel: ["ReadData: Rest" ("State(s) in Front (\"\")") "ReadData: Length" ("State(s) in Front (\"\")")] -> w353
          frame #0 {
            n152 = call <vilib>:"Merge Errors.vi"("error in 2 (no error)"=errorcluster {"status"=FALSE, "code"=7000, "source"="Message not for Me"}, "error in 1 (no error)"=w381) -> ("error out"=w379:errorcluster)  [unwired: 5 in]
          }
          frame #1 {
          }
        }
        n153 = call <vilib>:"Add State(s) to Queue__jki_lib_state_machine.vi"("State(s) in Front (\"\")"=w353, "State(s) in (\"\")"=w365) -> ("States Out"=w364:string)  [unwired: 13 in]
      }
      frame #26 {
        w398 = u8 224  # ESC
        # "Your code here.\n(You can make a copy of, or modify, this frame)"
        n154 = Unbundle By Name(w409) -> ("ComPort"=w392:refnum<visa-resource-name>, "ReadArray"=w390:u8[], "CRCArray"=w384:u8[])
        n155 = VISA Read(VISA resource name=w392, byte count=u32 1, error in (no error)=w404) -> (read buffer=w406:string, error out=w394:errorcluster)  [unwired: 2 out]
        n156 = String To Byte Array(string=w406) -> (unsigned byte array=w396:u8[])
        n157 = local write "ReadArray"(w390) -> ()
        n158 = Index Array(array=w396, index=0) -> (element=w400:u8)
        n159 = Equal?(x=w400, y=w398) -> (x = y?=w397:bool)
        n160 = case shown="False" w397 {
          tunnel: [w415 w416] -> w385
          tunnel: w396 -> [w415 w423]
          tunnel: [w414 w417] -> w395
          tunnel: w390 -> [w414 w424]
          tunnel: w394 -> [w413 w420]
          tunnel: [w413 w419] -> w393
          tunnel: w392 -> [_ w418]
          frame #0 {
          }
          frame #1 {
            n161 = VISA Read(VISA resource name=w418, byte count=u32 1, error in (no error)=w420) -> (read buffer=w422:string, error out=w419:errorcluster)  [unwired: 2 out]
            n162 = String To Byte Array(string=w422) -> (unsigned byte array=w416:u8[])
            n163 = Build Array (concatenate)(w424, w423) -> (w417:u8[])
          }
        }
        n164 = Index Array(array=w385, index=0) -> (element=w389:u8)
        n165 = Build Array (concatenate)(w395, w385) -> (w410:u8[])
        n166 = Subtract(x=w389, y=u8 6) -> (x-y=w387:u8)
        "element" <- w387
        n167 = Build Array (concatenate)(w384, w385) -> (w386:u8[])
        n168 = Less Or Equal?(x=w387, y=u8 0 ("0")) -> (x <= y?=w403:bool)
        n169 = Bundle By Name(cluster=w409, "ReadArray"=w410, "CRCArray"=w386, "Bytes Remaining"=w387) -> (w408:T3)
        n170 = case shown="False" w403 {
          tunnel: w393 -> [w426 w430]
          tunnel: [w426 w428] -> w402
          tunnel: ["ReadData: Bytes" ("State(s) in Front (\"\")") "ReadData: Rest" ("State(s) in Front (\"\")")] -> w401
          frame #0 {
          }
          frame #1 {
            n171 = call <vilib>:"Merge Errors.vi"("error in 2 (no error)"=errorcluster {"status"=FALSE, "code"=7000, "source"="0 Length"}, "error in 1 (no error)"=w430) -> ("error out"=w428:errorcluster)  [unwired: 5 in]
          }
        }
        n172 = call <vilib>:"Add State(s) to Queue__jki_lib_state_machine.vi"("State(s) in Front (\"\")"=w401, "State(s) in (\"\")"=w412) -> ("States Out"=w411:string)  [unwired: 13 in]
      }
      frame #27 {
        w444 = u8 224  # ESC
        # "Your code here.\n(You can make a copy of, or modify, this frame)"
        n173 = Unbundle By Name(w453) -> ("ComPort"=w438:refnum<visa-resource-name>, "ReadArray"=w434:u8[], "Bytes Remaining"=w436:u8, "CRCArray"=w431:u8[])
        n174 = VISA Read(VISA resource name=w438, byte count=u32 1, error in (no error)=w449) -> (read buffer=w450:string, error out=w440:errorcluster)  [unwired: 2 out]
        n175 = String To Byte Array(string=w450) -> (unsigned byte array=w442:u8[])
        n176 = Index Array(array=w442, index=0) -> (element=w446:u8)
        n177 = Equal?(x=w446, y=w444) -> (x = y?=w443:bool)
        n178 = case shown="True" w443 {
          tunnel: [w459 w460] -> w433
          tunnel: w442 -> [w459 w467]
          tunnel: [w458 w461] -> w441
          tunnel: w434 -> [w458 w468]
          tunnel: w440 -> [w457 w464]
          tunnel: [w457 w463] -> w439
          tunnel: w438 -> [_ w462]
          frame #0 {
          }
          frame #1 {
            n179 = VISA Read(VISA resource name=w462, byte count=u32 1, error in (no error)=w464) -> (read buffer=w466:string, error out=w463:errorcluster)  [unwired: 2 out]
            n180 = String To Byte Array(string=w466) -> (unsigned byte array=w460:u8[])
            n181 = Build Array (concatenate)(w468, w467) -> (w461:u8[])
          }
        }
        n182 = local write "ReadArray"(w434) -> ()
        n183 = Decrement(x=w436) -> (x-1=w435:u8)
        n184 = Build Array (concatenate)(w431, w433) -> (w432:u8[])
        n185 = Build Array (concatenate)(w441, w433) -> (w454:u8[])
        n186 = Greater Than 0?(x=w435) -> (x > 0?=w437:bool)
        n187 = Bundle By Name(cluster=w453, "ReadArray"=w454, "CRCArray"=w432, "Bytes Remaining"=w435) -> (w452:T3)
        n188 = case shown="False" w437 {
          tunnel: w439 -> [w472 w474]
          tunnel: [w470 w474] -> w448
          tunnel: ["ReadData: CRC1" ("State(s) in Front (\"\")") "ReadData: Bytes" ("State(s) in Front (\"\")")] -> w447
          frame #0 {
            n189 = call <vilib>:"Merge Errors.vi"("error in 2 (no error)"=errorcluster {"status"=FALSE, "code"=7000, "source"="0 Length"}, "error in 1 (no error)"=w472) -> ("error out"=w470:errorcluster)  [unwired: 5 in]
          }
          frame #1 {
          }
        }
        n190 = call <vilib>:"Add State(s) to Queue__jki_lib_state_machine.vi"("State(s) in Front (\"\")"=w447, "State(s) in (\"\")"=w456) -> ("States Out"=w455:string)  [unwired: 13 in]
      }
      frame #28 {
        w483 = u8 224  # ESC
        # "Your code here.\n(You can make a copy of, or modify, this frame)"
        n191 = Unbundle By Name(w491) -> ("ComPort"=w477:refnum<visa-resource-name>, "ReadArray"=w479:u8[])
        n192 = VISA Read(VISA resource name=w477, byte count=u32 1, error in (no error)=w487) -> (read buffer=w488:string, error out=w478:errorcluster)  [unwired: 2 out]
        n193 = String To Byte Array(string=w488) -> (unsigned byte array=w481:u8[])
        n194 = Index Array(array=w481, index=0) -> (element=w485:u8)
        n195 = Equal?(x=w485, y=w483) -> (x = y?=w482:bool)
        n196 = case shown="False" w482 {
          tunnel: [w497 w498] -> w476
          tunnel: w481 -> [w497 w505]
          tunnel: [w496 w499] -> w480
          tunnel: w479 -> [w496 w506]
          tunnel: w478 -> [w495 w502]
          tunnel: [w495 w501] -> w475
          tunnel: w477 -> [_ w500]
          frame #0 {
          }
          frame #1 {
            n197 = VISA Read(VISA resource name=w500, byte count=u32 1, error in (no error)=w502) -> (read buffer=w504:string, error out=w501:errorcluster)  [unwired: 2 out]
            n198 = String To Byte Array(string=w504) -> (unsigned byte array=w498:u8[])
            n199 = Build Array (concatenate)(w506, w505) -> (w499:u8[])
          }
        }
        n200 = Build Array (concatenate)(w480, w476) -> (w492:u8[])
        n201 = Bundle By Name(cluster=w491, "ReadArray"=w492, "CRCRead"=w476) -> (w490:T3)
        n202 = call <vilib>:"Add State(s) to Queue__jki_lib_state_machine.vi"("State(s) in Front (\"\")"="ReadData: CRC2" ("State(s) in Front (\"\")"), "State(s) in (\"\")"=w494) -> ("States Out"=w493:string)  [unwired: 13 in]
      }
      frame #29 {
        w518 = u8 224  # ESC
        # "Your code here.\n(You can make a copy of, or modify, this frame)"
        n203 = Unbundle By Name(w526) -> ("ComPort"=w513:refnum<visa-resource-name>, "ReadArray"=w509:u8[], "CRCRead"=w508:u8[])
        n204 = VISA Read(VISA resource name=w513, byte count=u32 1, error in (no error)=w522) -> (read buffer=w523:string, error out=w514:errorcluster)  [unwired: 2 out]
        n205 = String To Byte Array(string=w523) -> (unsigned byte array=w516:u8[])
        n206 = Index Array(array=w516, index=0) -> (element=w520:u8)
        n207 = Equal?(x=w520, y=w518) -> (x = y?=w517:bool)
        n208 = case shown="True" w517 {
          tunnel: [w531 w532] -> w510
          tunnel: w516 -> [w531 w539]
          tunnel: [w530 w533] -> w515
          tunnel: w509 -> [w530 w540]
          tunnel: w514 -> [w529 w536]
          tunnel: [w529 w535] -> w512
          tunnel: w513 -> [_ w534]
          frame #0 {
          }
          frame #1 {
            n209 = VISA Read(VISA resource name=w534, byte count=u32 1, error in (no error)=w536) -> (read buffer=w538:string, error out=w535:errorcluster)  [unwired: 2 out]
            n210 = String To Byte Array(string=w538) -> (unsigned byte array=w532:u8[])
            n211 = Build Array (concatenate)(w540, w539) -> (w533:u8[])
          }
        }
        n212 = local write "ReadArray"(w509) -> ()
        n213 = Build Array (concatenate)(w515, w510) -> (w511:u8[])
        n214 = Build Array (concatenate)(w508, w510) -> (w507:u8[])
        n215 = Bundle By Name(cluster=w526, "ReadArray"=w511, "CRCRead"=w507) -> (w525:T3)
        n216 = local write "CRCRead"(w507) -> ()
        n217 = call <vilib>:"Add State(s) to Queue__jki_lib_state_machine.vi"("State(s) in Front (\"\")"="ReadData: CheckCRC" ("State(s) in Front (\"\")"), "State(s) in (\"\")"=w528) -> ("States Out"=w527:string)  [unwired: 13 in]
      }
      frame #30 {
        # "Your code here.\n(You can make a copy of, or modify, this frame)"
        n218 = Unbundle By Name(w543) -> ("CRCRead"=w547:u8[], "CRCArray"=w542:u8[])
        "DataReturned" <- w542
        n219 = call "crc16-ccitt (x1021).vi"("error in (no error)"=w548, "unsigned byte array"=w542) -> ("error out (dup)"=w544:errorcluster, "CRC"=w541:u8[])  [unwired: 8 in]
        n220 = Equal?(x=w547, y=w541) -> (x = y?=w546:bool)
        "CRC Match" <- w546
        n221 = local write "CRC Calc"(w541) -> ()
        n222 = case shown="True" w546 {
          tunnel: ["ReadData: Rest" ("State(s) in Front (\"\")") "ReadData: ETX" ("State(s) in Front (\"\")")] -> w549
          tunnel: [w552 w556] -> w545
          tunnel: w544 -> [w554 w556]
          frame #0 {
            n223 = call <vilib>:"Merge Errors.vi"("error in 2 (no error)"=errorcluster {"status"=FALSE, "code"=7000, "source"="CRC No Match"}, "error in 1 (no error)"=w554) -> ("error out"=w552:errorcluster)  [unwired: 5 in]
          }
          frame #1 {
          }
        }
        n224 = call <vilib>:"Add State(s) to Queue__jki_lib_state_machine.vi"("State(s) in Front (\"\")"=w549, "State(s) in (\"\")"=w551) -> ("States Out"=w550:string)  [unwired: 13 in]
      }
      frame #31 {
        w558 = u8 226  # STX
        # "Your code here.\n(You can make a copy of, or modify, this frame)"
        n225 = Unbundle By Name(w570) -> ("ComPort"=w573:refnum<visa-resource-name>, "ReadArray"=w572:u8[])
        n226 = VISA Read(VISA resource name=w573, byte count=u32 1, error in (no error)=w568) -> (read buffer=w562:string, error out=w566:errorcluster)  [unwired: 2 out]
        n227 = String To Byte Array(string=w562) -> (unsigned byte array=w561:u8[])
        n228 = Index Array(array=w561, index=0) -> (element=w559:u8)
        n229 = Build Array (concatenate)(w572, w561) -> (w571:u8[])
        n230 = Equal?(x=w559, y=w558) -> (x = y?=w567:bool)
        n231 = Bundle By Name(cluster=w570, "ReadArray"=w571) -> (w569:T3)
        n232 = case shown="False" w567 {
          tunnel: w566 -> [w579 w581]
          tunnel: [w577 w581] -> w565
          tunnel: ["ReadData: Rest" ("State(s) in Front (\"\")") "ReadData: Destination" ("State(s) in Front (\"\")")] -> w564
          frame #0 {
            n233 = call <vilib>:"Merge Errors.vi"("error in 2 (no error)"=errorcluster {"status"=TRUE, "code"=7000, "source"="No STX"}, "error in 1 (no error)"=w579) -> ("error out"=w577:errorcluster)  [unwired: 5 in]
          }
          frame #1 {
          }
        }
        n234 = call <vilib>:"Add State(s) to Queue__jki_lib_state_machine.vi"("State(s) in Front (\"\")"=w564, "State(s) in (\"\")"=w575) -> ("States Out"=w574:string)  [unwired: 13 in]
      }
      frame #32 {
        w582 = u8 227  # ETX
        # "Your code here.\n(You can make a copy of, or modify, this frame)"
        n235 = Unbundle By Name(w594) -> ("ComPort"=w597:refnum<visa-resource-name>, "ReadArray"=w596:u8[])
        n236 = VISA Read(VISA resource name=w597, byte count=u32 1, error in (no error)=w592) -> (read buffer=w586:string, error out=w590:errorcluster)  [unwired: 2 out]
        n237 = String To Byte Array(string=w586) -> (unsigned byte array=w585:u8[])
        n238 = Index Array(array=w585, index=0) -> (element=w583:u8)
        n239 = Build Array (concatenate)(w596, w585) -> (w595:u8[])
        n240 = Equal?(x=w583, y=w582) -> (x = y?=w591:bool)
        n241 = Bundle By Name(cluster=w594, "ReadArray"=w595) -> (w593:T3)
        n242 = case shown="True" w591 {
          tunnel: w590 -> [w603 w605]
          tunnel: [w601 w605] -> w589
          tunnel: ["ReadData: Rest" ("State(s) in Front (\"\")") "ReadData: SendACK" ("State(s) in Front (\"\")")] -> w588
          frame #0 {
            n243 = call <vilib>:"Merge Errors.vi"("error in 2 (no error)"=errorcluster {"status"=TRUE, "code"=7000, "source"="No ETX"}, "error in 1 (no error)"=w603) -> ("error out"=w601:errorcluster)  [unwired: 5 in]
          }
          frame #1 {
          }
        }
        n244 = call <vilib>:"Add State(s) to Queue__jki_lib_state_machine.vi"("State(s) in Front (\"\")"=w588, "State(s) in (\"\")"=w599) -> ("States Out"=w598:string)  [unwired: 13 in]
      }
      frame #33 {
        n245 = Unbundle By Name(w608) -> ("ComPort"=w610:refnum<visa-resource-name>, "ReadArray"=w609:u8[])
        n246 = while {
          shift-right: [w615] -> w606
          shift-left: w609 -> [w617]
          tunnel: w610 -> [w616]
          stop <- w614 stop-if-true
          n247 = VISA Read(VISA resource name=w616, byte count=u32 1) -> (read buffer=w619:string, error out=w614:errorcluster)  [unwired: 1 in, 2 out]
          n248 = String To Byte Array(string=w619) -> (unsigned byte array=w618:u8[])
          n249 = Build Array (concatenate)(w617, w618) -> (w615:u8[])
        }
        n250 = Bundle By Name(cluster=w608, "ReadArray"=w606) -> (w607:T3)
        n251 = call <vilib>:"Add State(s) to Queue__jki_lib_state_machine.vi"("State(s) in (\"\")"=w613) -> ("States Out"=w612:string)  [unwired: 14 in]
      }
      frame #34 {
        w624 = u8 225  # ACK
        n252 = Unbundle By Name(w633) -> ("ComPort"=w632:refnum<visa-resource-name>)
        n253 = Build Array(w624) -> (w628:u8[])
        n254 = Byte Array To String(unsigned byte array=w628) -> (string=w626:string)
        n255 = VISA Write(VISA resource name=w632, write buffer=w626, error in (no error)=w631) -> (VISA resource name out=w630:refnum<visa-resource-name>, error out=w625:errorcluster)  [unwired: 1 out]
        n256 = VISA Read(VISA resource name=w630, byte count=u32 1, error in (no error)=w625) -> (read buffer=w627:string, error out=w622:errorcluster)  [unwired: 2 out]
        n257 = Equal?(x=w626, y=w627) -> (x = y?=w621:bool)
        "ACK" <- w621
        n258 = case shown="False" w621 {
          tunnel: [w638 w641] -> w623
          tunnel: w622 -> [w636 w639]
          frame #0 {
            n259 = call <vilib>:"Merge Errors.vi"("error in 2 (no error)"=errorcluster {"status"=FALSE, "code"=0, "source"="ACKed"} ("error in 1 (no error)"), "error in 1 (no error)"=w636) -> ("error out"=w638:errorcluster)  [unwired: 5 in]
          }
          frame #1 {
            n260 = call <vilib>:"Merge Errors.vi"("error in 2 (no error)"=errorcluster {"status"=FALSE, "code"=0, "source"="ACKed Bad"} ("error in 1 (no error)"), "error in 1 (no error)"=w639) -> ("error out"=w641:errorcluster)  [unwired: 5 in]
          }
        }
        n261 = call <vilib>:"Add State(s) to Queue__jki_lib_state_machine.vi"("State(s) in (\"\")"=w635) -> ("States Out"=w634:string)  [unwired: 14 in]
      }
    }
    n262 = flat-sequence {
      tunnel: w8 -> [w14]
      frame #0 {
        "States Out" <- w14
      }
    }
    "error out" <- w3
  }
